vi "HT3_Test.vi"() -> ()   [LabVIEW 2009]
panel:
  out "Image Header":T1
  out "Stop After (ms)":i32
  out "Stop Reason":enum16{"timeover", "manual", "overflow"}(ring)
  out "Num Records":i32
  out "Header":T2
  out "error out":errorcluster
  in  "error in":errorcluster
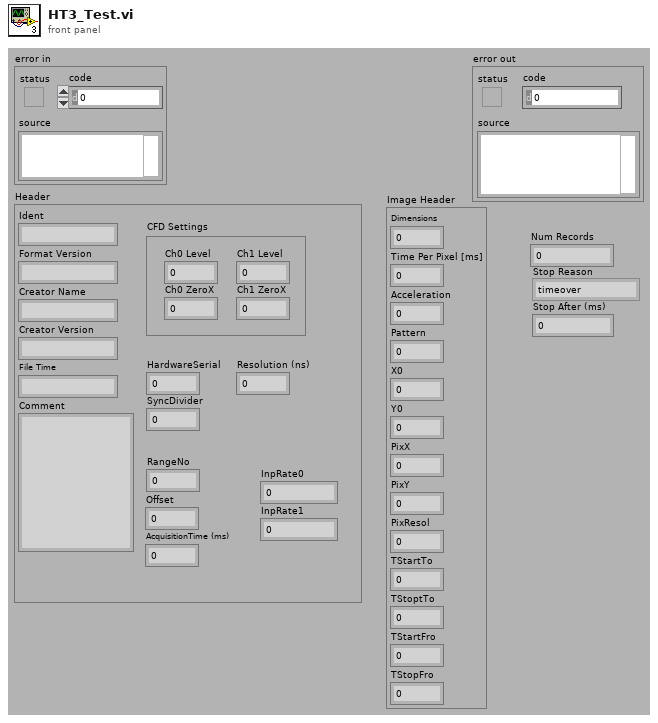
[diagram p1: front panel]
types:
  T1 = cluster{"Dimensions":i32, "Time Per Pixel [ms]":dbl, "Acceleration":i32, "Pattern":i32, "X0":sgl, "Y0":sgl, "PixX":i32, "PixY":i32, "PixResol":sgl, "TStartTo":sgl, "TStoptTo":sgl, "TStartFro":sgl, "TStopFro":sgl}
  T2 = cluster{"Ident":string, "Format Version":string, "Creator Name":string, "Creator Version":string, "File Time":string, "Comment":string, "RangeNo":i32, "Offset":i32, "AcquisitionTime (ms)":i32, "HardwareSerial":i32, "SyncDivider":i32, "Resolution (ns)":sgl, "CFD Settings":cluster{"Ch0 Level":i32, "Ch0 ZeroX":i32, "Ch1 Level":i32, "Ch1 ZeroX":i32}, "InpRate0":i32, "InpRate1":i32}
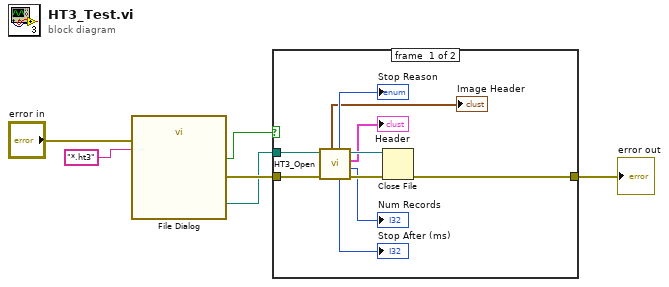
[diagram p0: block diagram]
diagram:
  n1 = call "File Dialog"("error in"="error in", "pattern (all files)"="*.ht3") -> ("selected path"=w4:path, "cancelled"=w3:bool, "error out"=w5:errorcluster)  [unwired: 5 in, 6 out]
  n2 = case shown="False" w3 {
    tunnel: w5 -> [w16 w17]
    tunnel: w4 -> [w15 _]
    tunnel: [w12 w17] -> w2
    frame #0 {
      n3 = call "HT3_Open.vi"("error in"=w16, "File Path"=w15) -> ("error out"=w13:errorcluster, "Num Records"=→"Num Records":i32, "Header"=→"Header":T2, "refnum out"=w14:refnum<file>, "Stop After (ms)"=→"Stop After (ms)":i32, "Stop Reason"=→"Stop Reason":enum16{"timeover", "manual", "overflow"}, "Image Header"=→"Image Header":T1)  [unwired: 3 out]
      n4 = Close File(refnum=w14, error in=w13) -> (error out=w12:errorcluster)  [unwired: 1 out]
    }
    frame #1 {
    }
  }
  "error out" <- w2
